vi "Create Body.vi"(6 "Draw Mode":T8(ring)=enum."Triangles", 7 "3D Comet Property":T4={"General Property"={"Plot Name"="", "Coordinate System"=enum."Cartesian", "Opacity"=0.0}, "Projection Property"={"Draw XY"=FALSE, "Draw YZ"=FALSE, "Draw XZ"=FALSE}, "Plot Property"={"Sprite Type"=enum."Empty Square", "Point Size"=0.0, "Point Color"=0, "Line Style"=enum."None", "Line Width"=0.0, "Line Color"=0, "Antialiasing"=FALSE}, "Comet Property"={"Body length"=0.0}}, 8 "error in (no error)":errorcluster, 9 "Actual Transform In":T7, 10 "Plot Representation In":T1, 11 "Plot Object In":refnum<vi>) -> (0 "error out":errorcluster, 1 "Actual Transform Out":T7, 2 "Plot Representation Out":T1, 3 "Plot Object Out":refnum<vi>, 4 "Track Object Out":refnum<vi>)   [LabVIEW 2020, in "3D Comet.lvclass"]
uses:
  <vilib>/Math Plots/3D Math Plots/3D Comet/3D Comet/3D Comet.lvclass
  <vilib>/Math Plots/3D Math Plots/3D Plot/3D Plot/Typedef/Actual Transform.ctl
  <vilib>/Math Plots/3D Math Plots/3D Plot/3D Plot/Typedef/Range Clusters.ctl
  <vilib>/Math Plots/3D Math Plots/3D Plot/3D Plot/Typedef/Plot Representation.ctl
  <vilib>/Math Plots/3D Math Plots/3D Plot/3D Plot/Typedef/Mesh Data.ctl
  <vilib>/Math Plots/3D Math Plots/3D Comet/3D Comet/Typedef/3D Comet Property.ctl
  <vilib>/Math Plots/3D Math Plots/3D Plot/3D Plot/Typedef/Sprite Type.ctl
  <vilib>/Math Plots/3D Math Plots/3D Plot/3D Plot/Typedef/Line Type.ctl
  <vilib>/Utility/miscctls.llb/LV3DPointTypeDef.ctl
  <vilib>/picture/3D Picture Control/NI_3D Picture Control.lvlib
  <vilib>/Math Plots/3D Math Plots/3D Plot/3D Plot/3D Plot.lvclass
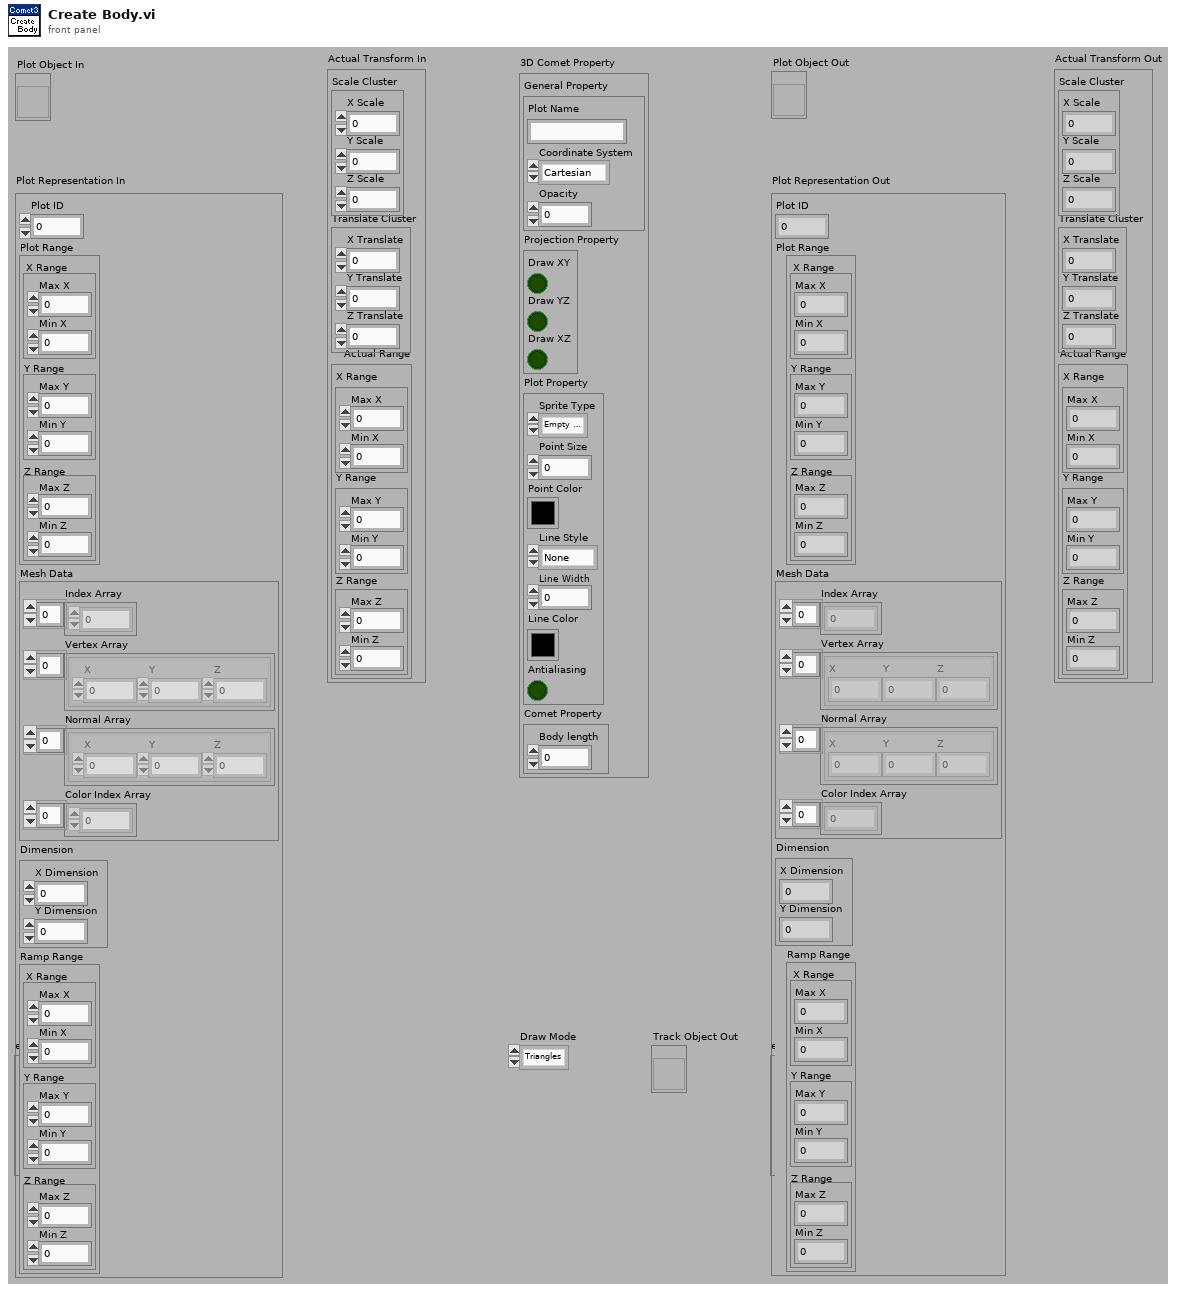
[diagram p1: front panel]
types:
  T1 = typedef "3D Plot.lvclass/Plot Representation.ctl" = cluster{"Plot ID":i32, "Plot Range":T2, "Mesh Data":T3, "Dimension":cluster{"X Dimension":i32, "Y Dimension":i32}, "Ramp Range":T2}
  T2 = typedef "3D Plot.lvclass/Range Clusters.ctl" = cluster{"X Range":cluster{"Max X":sgl, "Min X":sgl}, "Y Range":cluster{"Max Y":sgl, "Min Y":sgl}, "Z Range":cluster{"Max Z":sgl, "Min Z":sgl}}
  T3 = typedef "3D Plot.lvclass/Mesh Data.ctl" = cluster{"Index Array":u32[], "Vertex Array":cluster{"X":sgl, "Y":sgl, "Z":sgl}[], "Normal Array":cluster{"X":sgl, "Y":sgl, "Z":sgl}[], "Color Index Array":i32[]}
  T4 = typedef "3D Comet.lvclass/3D Comet Property.ctl" = cluster{"General Property":cluster{"Plot Name":string, "Coordinate System":enum16{"Cartesian", "Cylindrical", "Spherical"}, "Opacity":sgl}, "Projection Property":cluster{"Draw XY":bool, "Draw YZ":bool, "Draw XZ":bool}, "Plot Property":cluster{"Sprite Type":T5, "Point Size":sgl, "Point Color":u32, "Line Style":T6, "Line Width":sgl, "Line Color":u32, "Antialiasing":bool}, "Comet Property":cluster{"Body length":sgl}}
  T5 = typedef "3D Plot.lvclass/Sprite Type.ctl" = enum16{"None", "Empty Square", "Solid Square", "Empty Diamond", "Solid Diamond", "Empty Circle", "Solid Circle", "Asterisk", "Bold X", "Wireframe Sphere", "Solid Sphere", "Wireframe Cube", "Solid Cube"}
  T6 = typedef "3D Plot.lvclass/Line Type.ctl" = enum16{"None", "Solid", "Dash", "Dot", "Dash Dot"}
  T7 = typedef "3D Plot.lvclass/Actual Transform.ctl" = cluster{"Scale Cluster":cluster{"X Scale":sgl, "Y Scale":sgl, "Z Scale":sgl}, "Translate Cluster":cluster{"X Translate":sgl, "Y Translate":sgl, "Z Translate":sgl}, "Actual Range":T2}
  T8 = enum16{"Points", "Lines", "Line Strip", "Line Loop", "Triangles", "Triangle Strip", "Triangle Fan", "Quads", "Quad Strip", "Polygon"}
  T9 = typedef "LV3DPointTypeDef.ctl" = cluster{"X":sgl, "Y":sgl, "Z":sgl}
  T10 = enum16{"Overall", "Per Primitive", "Per Vertex", "Binding Off"}
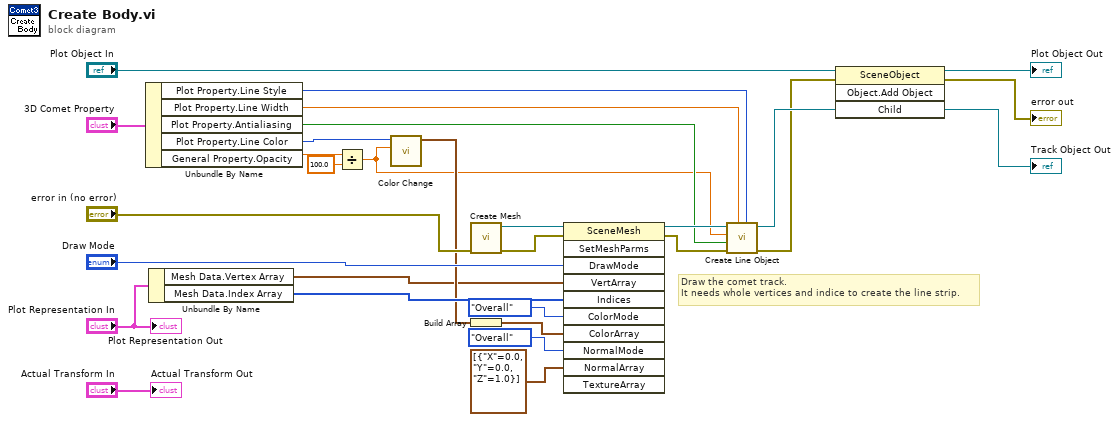
[diagram p0: block diagram]
diagram:
  # "Draw the comet track.\nIt needs whole vertices and indice to create the line strip."
  n1 = Unbundle By Name("3D Comet Property") -> ("Plot Property.Line Style"=w5:T6, "Plot Property.Line Width"=w6:sgl, "Plot Property.Antialiasing"=w3:bool, "Plot Property.Line Color"=w17:u32, "General Property.Opacity"=w4:sgl)
  n2 = Unbundle By Name("Plot Representation In") -> ("Mesh Data.Vertex Array"=w13:cluster{"X":sgl, "Y":sgl, "Z":sgl}[], "Mesh Data.Index Array"=w21:u32[])
  n3 = Divide(x=w4, y=sgl 100.0) -> (x/y=w2:sgl)
  n4 = call <vilib>:"Color Change.vi"("Alpha"=w2, "Color"=w17) -> ("RGBA"=w16:cluster{"R":sgl, "G":sgl, "B":sgl, "A":sgl})  [unwired: 9 out]
  n5 = call <vilib>:"Create Mesh.vi"("error in (no error)"="error in (no error)") -> ("error out"=w19:errorcluster, "New Mesh Refnum"=w22:refnum<vi>)  [unwired: 9 out]
  n6 = Build Array(w16) -> (w15:cluster{"R":sgl, "G":sgl, "B":sgl, "A":sgl}[])
  n7 = invoke class="SceneMesh" method="SetMeshParms"(reference=w22, error in=w19, "DrawMode"="Draw Mode", "VertArray"=w13, "Indices"=w21, "ColorMode"=T10."Overall" ("Color Binding Mode"), "ColorArray"=w15, "NormalMode"=T10."Overall" ("Normal Binding Mode"), "NormalArray"=T9[] [{"X"=0.0, "Y"=0.0, "Z"=1.0}] ("Normal Array")) -> (reference out=w10:refnum<vi>, error out=w11:errorcluster)  [unwired: 2 in, 9 out]
  n8 = call <vilib>:"Create Line Object.vi"("Line Style"=w5, "Line Width"=w6, "error in (no error)"=w11, "Antialiasing"=w3, "Alpha"=w2, "Mesh Ref In"=w10) -> ("error out"=w8:errorcluster, "Object Ref Out"=w9:refnum<vi>)  [unwired: 4 out]
  n9 = invoke class="SceneObject" method="Object.Add Object"(reference="Plot Object In", error in=w8, "Child"=w9) -> (reference out=→"Plot Object Out":refnum<vi>, error out=→"error out":errorcluster, "Child"=→"Track Object Out":refnum<vi>)  [unwired: 1 in, 1 out]
  "Actual Transform Out" <- "Actual Transform In"
  "Plot Representation Out" <- "Plot Representation In"
